vi "Combined Simulation VI v5.31.vi"(0 "Boondoggle Input":dbl) -> (1 "Rig Temperatures Cluster":T2, 2 "Line Data (Array of Clusters)":T1(array[cluster]))   [LabVIEW 2018]
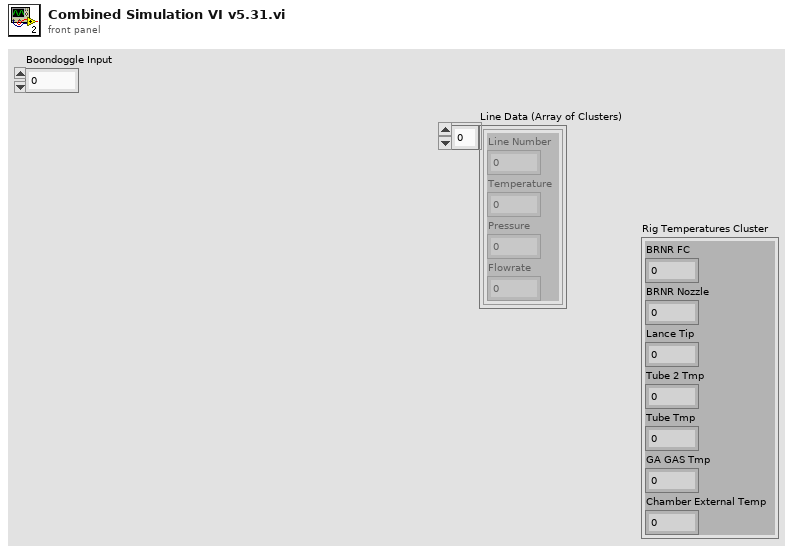
[diagram p1: front panel]
types:
  T1 = cluster{"Line Number":dbl, "Temperature":dbl, "Pressure":dbl, "Flowrate":dbl}[]
  T2 = cluster{"BRNR FC":dbl, "BRNR Nozzle":dbl, "Lance Tip":dbl, "Tube 2 Tmp":dbl, "Tube Tmp":dbl, "GA GAS Tmp":dbl, "Chamber External Temp":dbl}
  T3 = cluster{"Line Number":dbl, "Temperature":dbl, "Pressure":dbl, "Flowrate":dbl}
  T4 = cluster{"[0]":dbl, "[1]":dbl, "[2]":dbl, "[3]":dbl}
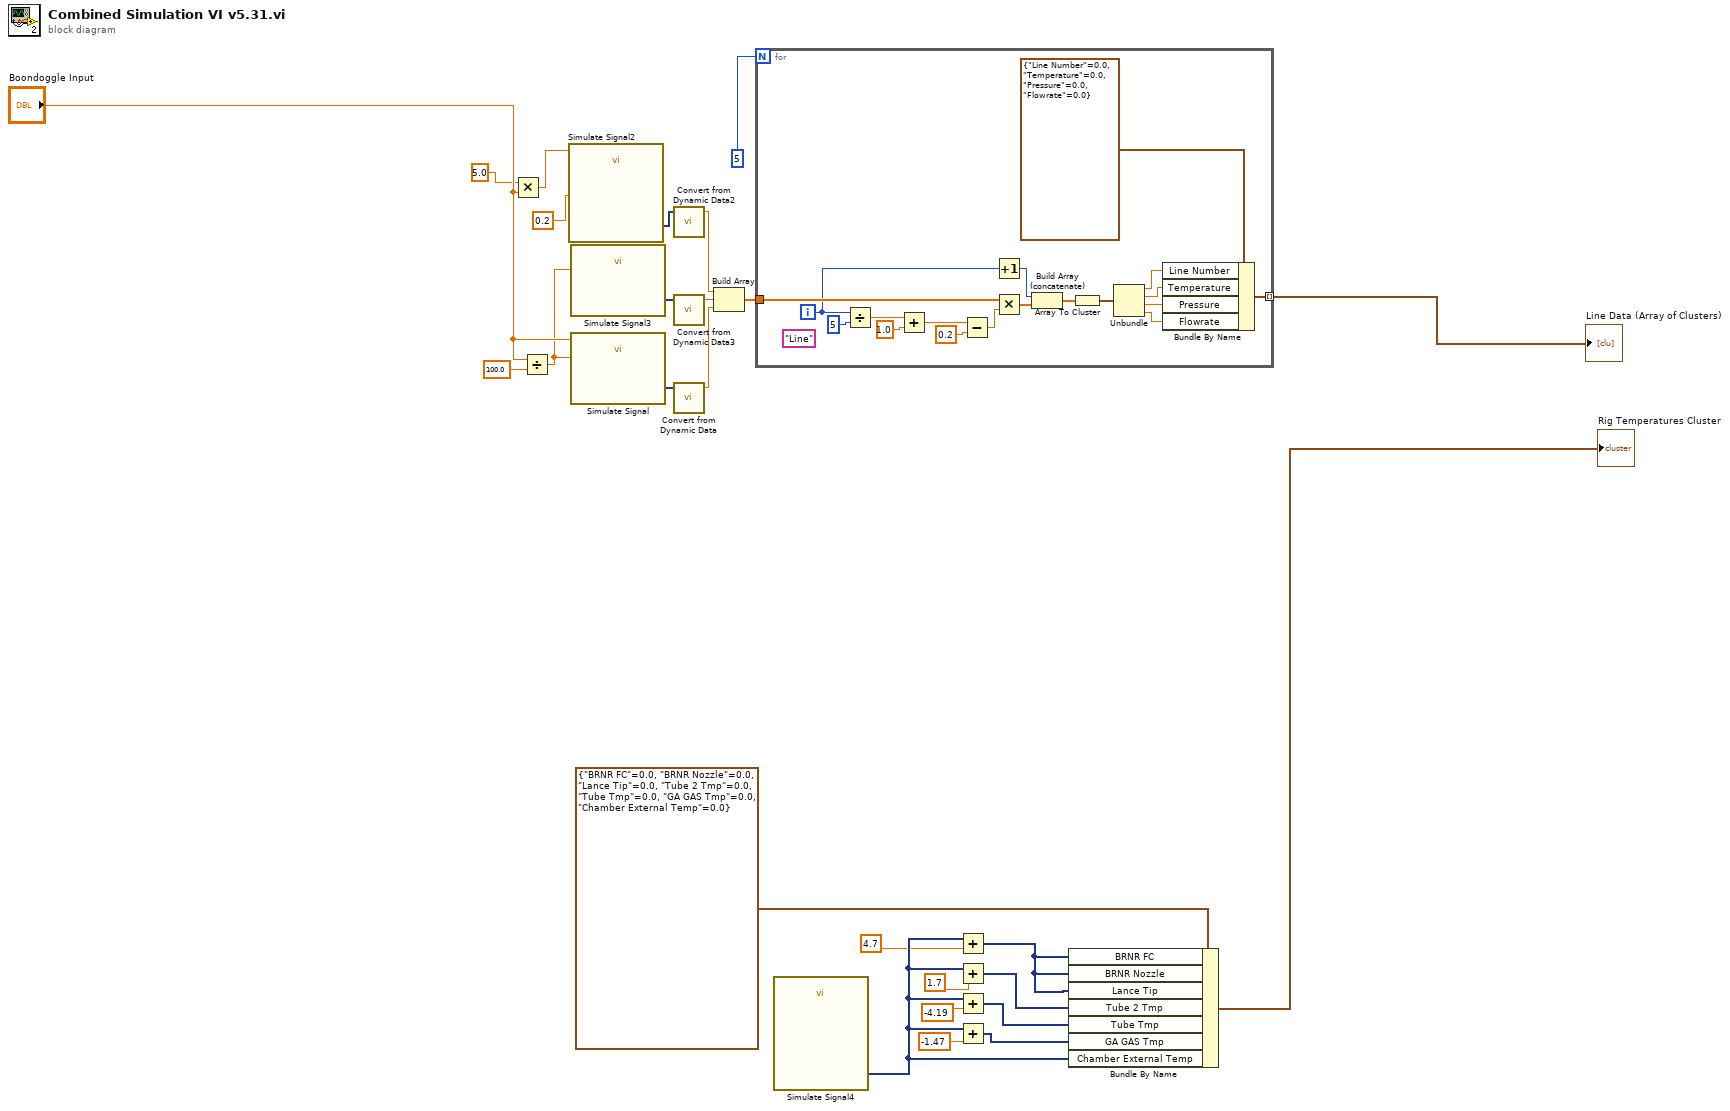
[diagram p0: block diagram]
diagram:
  n1 = Multiply(x=5.0 ("Offset"), y="Boondoggle Input") -> (x*y=w15:dbl)
  n2 = Divide(x="Boondoggle Input", y=100.0) -> (x/y=w12:dbl)
  n3 = call "Simulate Signal2"("Offset"=w15, "Spectral amplitude"=0.2) -> ("DC Temperature Signal"=w4:dynamicdata)  [unwired: 12 in, 1 out]
  n4 = call "Simulate Signal3"("Spectral amplitude"=w12) -> ("DC Pressure Signal"=w3:dynamicdata)  [unwired: 13 in, 1 out]
  n5 = call "Simulate Signal"("Offset"="Boondoggle Input", "Spectral amplitude"=w12) -> ("DC Flowrate Signal"=w5:dynamicdata)  [unwired: 12 in, 1 out]
  n6 = call "Convert from Dynamic Data2"("Dynamic Data Type"=w4) -> ("Scalar"=w6:dbl)  [unwired: 3 in]
  n7 = call "Convert from Dynamic Data3"("Dynamic Data Type"=w3) -> ("Scalar"=w7:dbl)  [unwired: 3 in]
  n8 = call "Convert from Dynamic Data"("Dynamic Data Type"=w5) -> ("Scalar"=w8:dbl)  [unwired: 3 in]
  n9 = Build Array(w6, w7, w8) -> (w10:dbl[])
  n10 = for {
    N: 5 -> [_]
    tunnel: w10 -> [w44]
    tunnel: [w30] -> w1 mode=indexing
    i -> [w28]
    (unwired) "Line"
    n11 = Divide(x=w28, y=5) -> (x/y=w42:dbl)
    n12 = Add(x=w42, y=1.0) -> (x+y=w40:dbl)
    n13 = Subtract(x=w40, y=0.2) -> (x-y=w38:dbl)
    n14 = Increment(x=w28) -> (x+1=w27:i32)
    n15 = Multiply(x=w44, y=w38) -> (x*y=w37:dbl[])
    n16 = Build Array (concatenate)(w27, w37) -> (w36:dbl[])
    n17 = Array To Cluster(array=w36) -> (cluster=w35:T4)
    n18 = Unbundle(w35) -> ("[0]"=w34:dbl, "[1]"=w33:dbl, "[2]"=w32:dbl, "[3]"=w31:dbl)
    n19 = Bundle By Name(cluster=T3 {"Line Number"=0.0, "Temperature"=0.0, "Pressure"=0.0, "Flowrate"=0.0}, "Line Number"=w34, "Temperature"=w33, "Pressure"=w32, "Flowrate"=w31) -> (w30:T3)
  }
  "Line Data (Array of Clusters)" <- w1
  n20 = call "Simulate Signal4"() -> ("Rig Temperatures"=w25:dynamicdata)  [unwired: 14 in, 1 out]
  n21 = Add(x=w25, y=4.7) -> (x+y=w17:dynamicdata)
  n22 = Add(x=w25, y=1.7) -> (x+y=w19:dynamicdata)
  n23 = Add(x=w25, y=-4.19) -> (x+y=w21:dynamicdata)
  n24 = Add(x=w25, y=-1.47) -> (x+y=w23:dynamicdata)
  n25 = Bundle By Name(cluster=T2 {"BRNR FC"=0.0, "BRNR Nozzle"=0.0, "Lance Tip"=0.0, "Tube 2 Tmp"=0.0, "Tube Tmp"=0.0, "GA GAS Tmp"=0.0, "Chamber External Temp"=0.0}, "BRNR FC"=w17, "BRNR Nozzle"=w17, "Lance Tip"=w17, "Tube 2 Tmp"=w19, "Tube Tmp"=w21, "GA GAS Tmp"=w23, "Chamber External Temp"=w25) -> (→"Rig Temperatures Cluster":T2)
